vi "SiCellDistMeasure.vi"() -> ()   [LabVIEW 2021]
uses:
  <vilib>/userDefined/High Color/IMAQdx.ctl
  include/GlobalVariables.vi
  Other Models/2010/Motion/AbortSingle.vi
  <vilib>/vision/driver/NI_Vision_Acquisition_Software.lvlib
panel:
  in  "AtEnd":string="G91\nG1 X-12.08 F100\nG90"
  out "error out":errorcluster
  out "XYZdist":string
  out "PrevY":dbl format="%#_13g"
  out "PrevX":dbl format="%#_13g"
  in  "Npoints":i32=14
  in  "NextPosition":string="G91\nG1 X12.08 F100\n//G1 X60.415F100"
  in  "TemplateFileName":string="C:\\Users\\TTUHEP\\Pictures\\Si_Y.png"
  out "CurrXYZdist":string
  in  "ObjectDetType":enum16{"Pattern", "ManualPick", "FidCircle"}(ring)
  in  "StartGCode":string="G90\n//G1 Z0 F100\nG1 X0.7942884\tY965.0350136 F100\rG1 Z75.0089"
  in  "StartPosition":enum16{"JoyStick", "FixedXY"}(ring)
  out "CamY":dbl
  out "CamX":dbl
  out "Radius":dbl
  out "CenterPosition":cluster{"X":sgl, "Y":sgl}
  in  "StopJoyStick":bool
  in  "Autofocus":T1={"Enable"=TRUE, "InitialStepSize"=0.05, "Tolerance"=0.02, "Abort"=FALSE} {"Tolerance" format="%#_13g"}
  out "Image":T2(plugin-control)
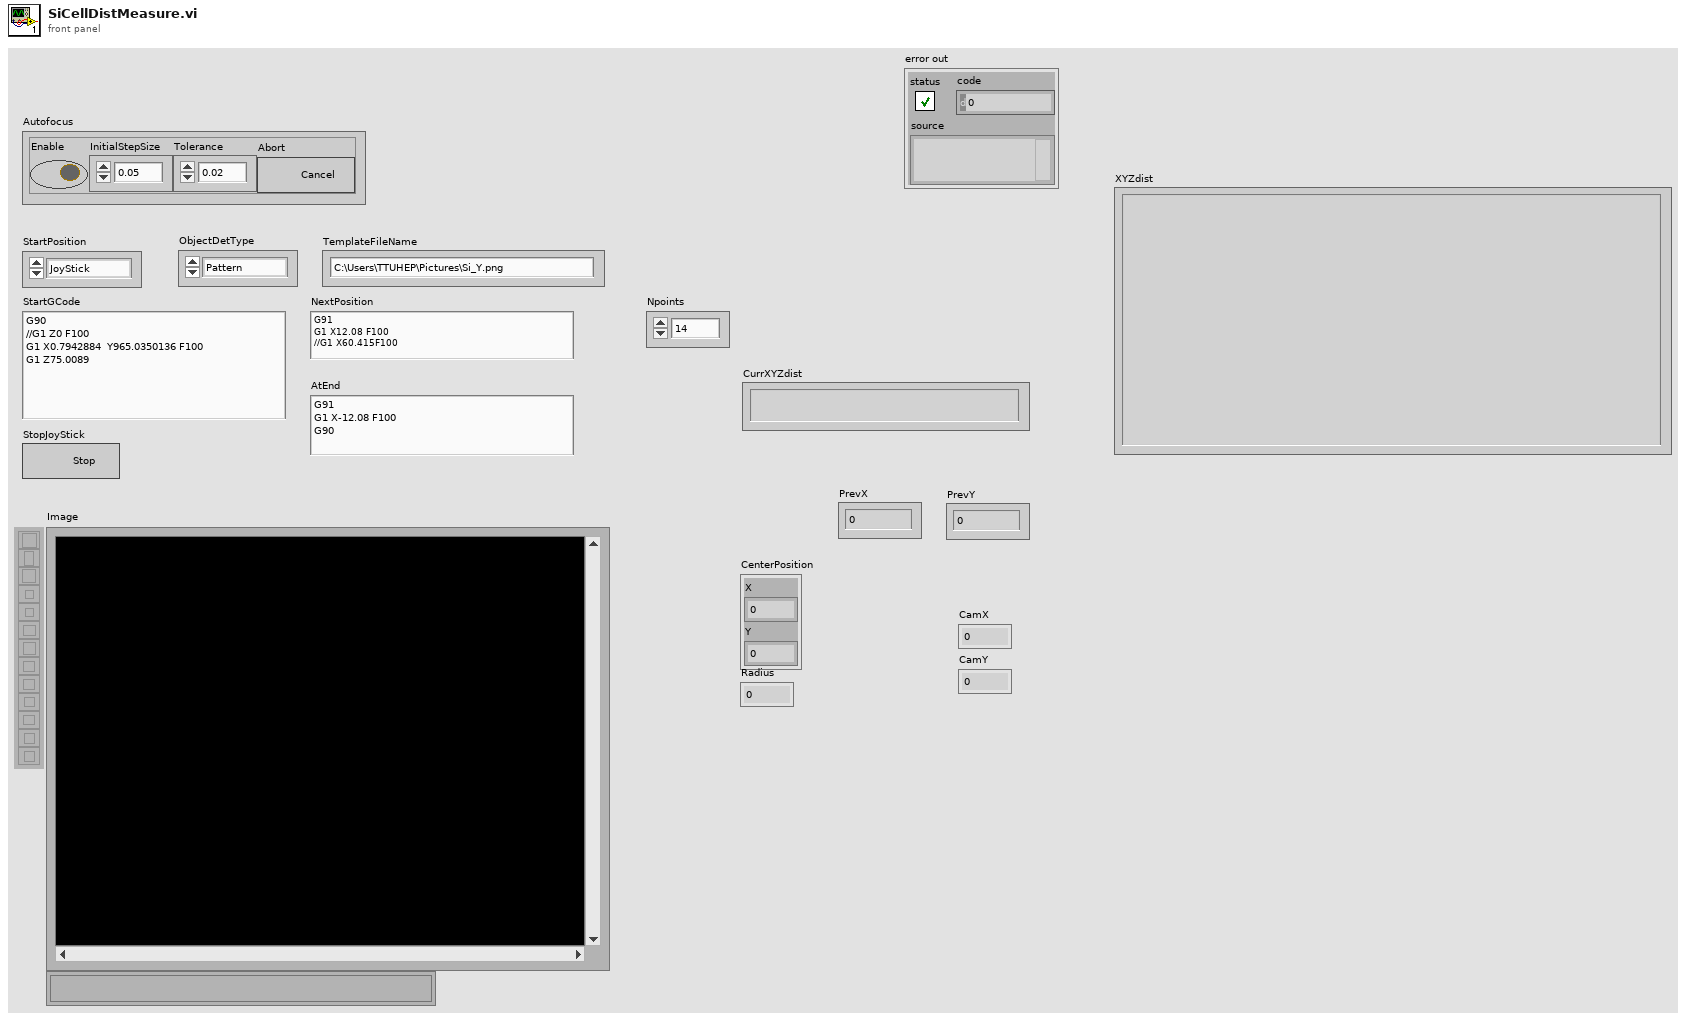
[diagram p1: front panel]
types:
  T1 = cluster{"Enable":bool, "InitialStepSize":dbl, "Tolerance":dbl, "Abort":bool}
  T2 = typedef "IMAQ Image.ctl" = refnum<image>
  T3 = typedef "IMAQdx.ctl" = refnum<k21>
  T4 = typedef "Image Type" = u32
  T5 = cluster{"Number of Matches Requested":i32, "Minimum Match Score":sgl, "Angle Ranges":cluster{"Start Angle":sgl, "End Angle":sgl}[]}
  T6 = typedef "IMAQ Point" = cluster{"X":sgl, "Y":sgl}
  T7 = cluster{"Position":cluster{"X":sgl, "Y":sgl}, "Radius":dbl, "Score":dbl}
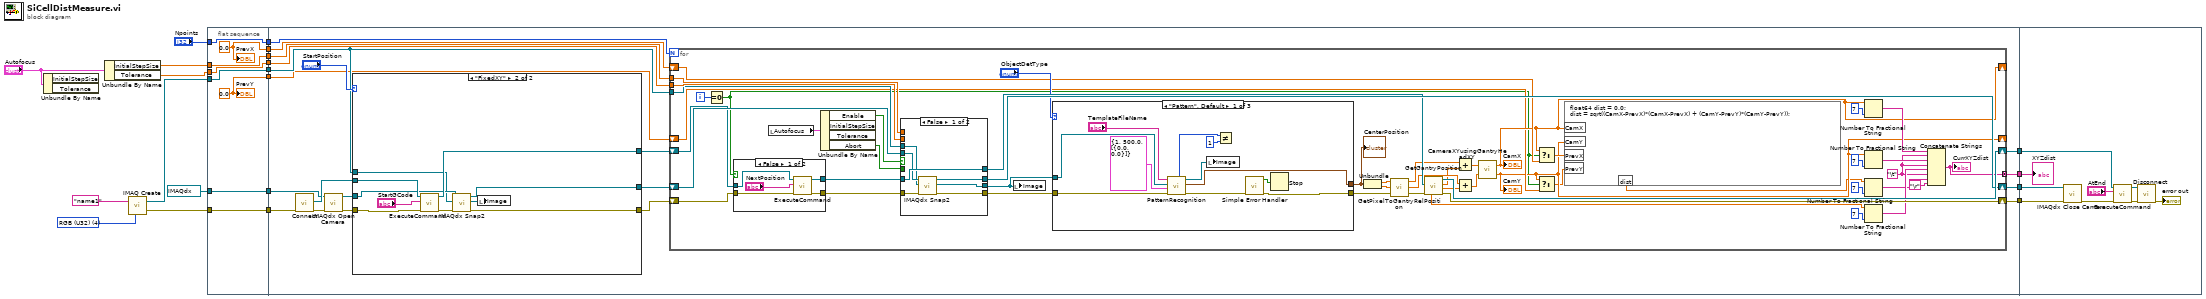
[diagram p0: block diagram]
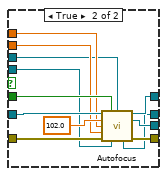
[diagram p3: hidden frame]
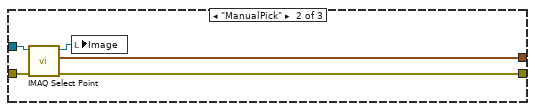
[diagram p4: hidden frame]
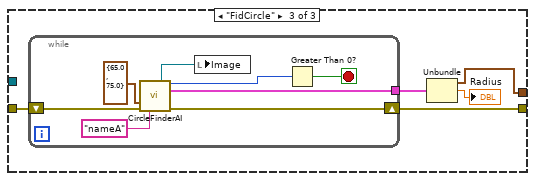
[diagram p5: hidden frame]
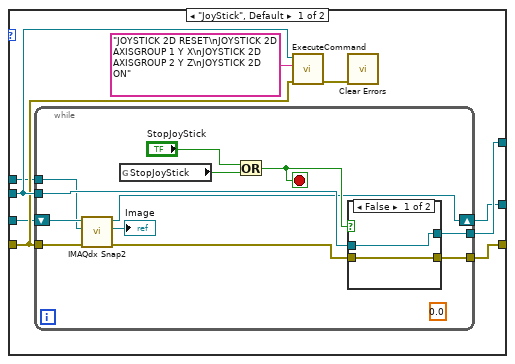
[diagram p6: hidden frame]
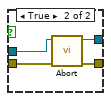
[diagram p7: hidden frame]
diagram:
  w15 = T4 4 items=["Grayscale (U8)", "Grayscale (I16)", "Grayscale (SGL)", "Complex (CSG)", "RGB (U32)", "HSL (U32)", "RGB (U64)", "Grayscale (U16)"] ("Image Type")
  n1 = Unbundle By Name("Autofocus") -> ()  [unwired: 2 out]
  n2 = Unbundle By Name("Autofocus") -> ("InitialStepSize"=w20:dbl, "Tolerance"=w21:dbl)
  n3 = call "IMAQ Create"("Image Name"="name1" ("ImageName"), "Image Type"=w15) -> ("New Image"=w14:T2, "error out"=w13:errorcluster)  [unwired: 3 in]
  n4 = flat-sequence {
    tunnel: "Npoints" -> [w24]
    tunnel: T3 "cam1" ("Camera") -> [w25]
    tunnel: w13 -> [w26]
    tunnel: w14 -> [w27]
    tunnel: w20 -> [w28]
    tunnel: w21 -> [w29]
    tunnel: [w29] -> w9
    tunnel: [w28] -> w8
    tunnel: [w27] -> w7
    tunnel: [w26] -> w6
    tunnel: [w25] -> w5
    tunnel: [w24] -> w4
    tunnel: [w23] -> w3
    tunnel: [w22] -> w2
    tunnel: [w45] -> w18
    tunnel: [w44] -> w17
    tunnel: [w38] -> w11
    tunnel: w9 -> [w49]
    tunnel: w8 -> [w48]
    tunnel: w7 -> [w41]
    tunnel: w6 -> [w42]
    tunnel: w5 -> [w40]
    tunnel: w4 -> [w36]
    tunnel: w3 -> [w33]
    tunnel: w2 -> [w32]
    tunnel: [w31] -> w1
    tunnel: w18 -> [w196]
    tunnel: w17 -> [w200]
    tunnel: w11 -> [w199]
    tunnel: w1 -> [w198]
    frame #0 {
      w22 = 0.0 ("PrevY")
      w23 = 0.0 ("PrevX")
      "PrevX" <- w23
      "PrevY" <- w22
    }
    frame #1 {
      n5 = call "Connect.vi"("error in (no error)"=w42) -> ("error out"=w46:errorcluster, "controller"=w47:refnum<k24>)  [unwired: 9 in]
      n6 = call <vilib>:"IMAQdx Open Camera.vi"("error in"=w46, "Session In"=w40) -> ("error out"=w39:errorcluster, "Session Out"=w30:T3)  [unwired: 8 in]
      n7 = case shown="\"FixedXY\"" "StartPosition" {
        tunnel: w47 -> [w162 w191]
        tunnel: [w160 w189] -> w35
        tunnel: w39 -> [w159 w190]
        tunnel: w41 -> [w158 w183]
        tunnel: w30 -> [w157 w187]
        tunnel: [w156 w185] -> w34
        tunnel: [w155 w184] -> w37
        frame "JoyStick", Default {
          n8 = while {
            tunnel: w162 -> [w175]
            tunnel: [w174] -> w156
            tunnel: [w173] -> w160
            tunnel: w159 -> [w169]
            shift-right: [w167] -> w155
            shift-left: w157 -> [w166]
            tunnel: w158 -> [w164]
            stop <- w170 stop-if-true
            (unwired) sgl 0.0 ("Rotate (degrees)")
            n9 = call <vilib>:"IMAQdx Snap2.vi"("error in"=w169, "Image In"=w164, "Session In"=w166) -> ("error out"=w165:errorcluster, "Image Out"=→"Image":T2, "Session Out"=w167:T3)  [unwired: 6 in]
            n10 = global read "GlobalVariables.vi" "StopJoyStick"() -> (w171:bool)
            n11 = Or(x="StopJoyStick", y=w171) -> (x .or. y?=w170:bool)
            n12 = case shown="False" w170 {
              tunnel: w175 -> [w177 w181]
              tunnel: w165 -> [w176 w180]
              tunnel: [w176 w179] -> w174
              tunnel: [w177 w178] -> w173
              frame False {
              }
              frame True {
                n13 = call-poly "Abort.vi"("error in (no error)"=w180, "controller in"=w181) -> ("error out"=w179:errorcluster, "controller out"=w178:refnum<k24>)  [unwired: 8 in]
              }
            }
          }
          n14 = call "ExecuteCommand.vi"("error in (no error)"=w159, "Command Code"="JOYSTICK 2D RESET\nJOYSTICK 2D AXISGROUP 1 Y X\nJOYSTICK 2D AXISGROUP 2 Y Z\nJOYSTICK 2D ON", "controller in"=w162) -> ("error out"=w161:errorcluster)  [unwired: 6 in, 2 out]
          n15 = call <vilib>:"Clear Errors.vi"("error in (no error)"=w161) -> ()  [unwired: 5 in, 2 out]
        }
        frame "FixedXY" {
          n16 = call "ExecuteCommand.vi"("error in (no error)"=w190, "Command Code"="StartGCode", "controller in"=w191) -> ("error out"=w186:errorcluster, "controller out"=w189:refnum<k24>)  [unwired: 6 in, 1 out]
          n17 = call <vilib>:"IMAQdx Snap2.vi"("error in"=w186, "Image In"=w183, "Session In"=w187) -> ("error out"=w185:errorcluster, "Image Out"=w182:T2, "Session Out"=w184:T3)  [unwired: 6 in]
          n18 = local write "Image"(w182) -> ()
        }
      }
      n19 = for {
        N: w36 -> [_]
        tunnel: w49 -> [w99]
        tunnel: w48 -> [w98]
        tunnel: w41 -> [w89]
        shift-right: [w97] -> w45
        shift-left: w35 -> [w53]
        shift-right: [w96] -> w44
        shift-left: w34 -> [w50]
        shift-right: [w88] -> w38
        shift-left: w37 -> [w71]
        shift-right: [w64] -> _
        shift-left: w33 -> [w65]
        shift-right: [w61] -> _
        shift-left: w32 -> [w63]
        tunnel: [w56] -> w31 mode=concatenating
        i -> [w66]
        w60 = "\t"
        n20 = Equal To 0?(x=w66) -> (x = 0?=w54:bool)
        n21 = case shown="False" w54 {
          tunnel: w53 -> [w103 w105]
          tunnel: [w102 w105] -> w52
          tunnel: [w101 w106] -> w51
          tunnel: w50 -> [w100 w106]
          frame False {
            n22 = call "ExecuteCommand.vi"("error in (no error)"=w100, "Command Code"="NextPosition", "controller in"=w103) -> ("error out"=w101:errorcluster, "controller out"=w102:refnum<k24>)  [unwired: 6 in, 1 out]
          }
          frame True {
          }
        }
        n23 = local read "Autofocus"() -> (w74:T1)
        n24 = Unbundle By Name(w74) -> ("Enable"=w73:bool, "Abort"=w72:bool)  [unwired: 2 out]
        n25 = case shown="False" w73 {
          tunnel: w99 -> [_ w121]
          tunnel: w98 -> [_ w122]
          tunnel: w52 -> [w113 w124]
          tunnel: [w107 w115] -> w87
          tunnel: [w113 w116] -> w86
          tunnel: w51 -> [w108 w120]
          tunnel: [w112 w117] -> w76
          tunnel: w72 -> [_ w125]
          tunnel: w89 -> [w109 w119]
          tunnel: w71 -> [w111 w118]
          tunnel: [w110 w114] -> w88
          frame False {
            n26 = call <vilib>:"IMAQdx Snap2.vi"("error in"=w108, "Image In"=w109, "Session In"=w111) -> ("error out"=w107:errorcluster, "Image Out"=w112:T2, "Session Out"=w110:T3)  [unwired: 6 in]
          }
          frame True {
            n27 = call "Autofocus.vi"("controller in"=w124, "AbortAutoFocus"=w125, "ImageIn"=w119, "SafeMaxZ"=102.0, "InitialStepSize"=w122, "Tolerance"=w121, "error in (no error)"=w120, "SessionIn"=w118) -> ("controller out"=w116:refnum<k24>, "Image"=w117:T2, "Session Out"=w114:T3, "error out"=w115:errorcluster)  [unwired: 2 in, 2 out]
          }
        }
        n28 = local write "Image"(w76) -> ()
        n29 = case shown="\"Pattern\", Default" "ObjectDetType" {
          tunnel: w87 -> [w132 w138 w146]
          tunnel: [w133 w140 w143] -> w85
          tunnel: [w127 w139 w142] -> w82
          tunnel: w76 -> [w135 w141 _]
          frame "Pattern", Default {
            n30 = call "PatternRecognition.vi"("error in (no error)"=w132, "MatchParameters"=T5 {"Number of Matches Requested"=1, "Minimum Match Score"=500.0, "Angle Ranges"=[{"Start Angle"=0.0, "End Angle"=0.0}]}, "ImageIn"=w135, "TemplateFileName"="TemplateFileName") -> ("error out"=w128:errorcluster, "Position"=w133:cluster{"x":sgl, "y":sgl}, "ImageFoundPattern"=w134:T2, "Number of Matches"=w130:i32)  [unwired: 2 in, 1 out]
            n31 = local write "Image"(w134) -> ()
            n32 = Not Equal?(x=w130, y=1) -> ()  [unwired: 1 out]
            n33 = call <vilib>:"Simple Error Handler.vi"("error in (no error)"=w128) -> ("error?"=w126:bool, "error out"=w127:errorcluster)  [unwired: 4 in, 3 out]
            n34 = Stop(stop? (T)=w126) -> ()
          }
          frame "ManualPick" {
            n35 = call "IMAQ Select Point"("error in (no error)"=w138, "Image In"=w141) -> ("error out"=w139:errorcluster, "Point"=w140:T6, "Image Out (duplicate)"=w137:T2)  [unwired: 6 in, 1 out]
            n36 = local write "Image"(w137) -> ()
          }
          frame "FidCircle" {
            n37 = while {
              tunnel: [w151] -> w145
              shift-right: [w150] -> w142
              shift-left: w146 -> [w152]
              stop <- w147 stop-if-true
              n38 = call "CircleFinderAI.vi"("Circle Descriptor"=cluster{"Min Radius":dbl, "Max Radius":dbl} {"Min Radius"=65.0, "Max Radius"=75.0}, "error in (no error)"=w152, "Image Name"="nameA") -> ("Image"=w149:T2, "NumCirclesFound"=w148:i32, "Circle0"=w151:T7, "error out"=w150:errorcluster)  [unwired: 7 in, 2 out]
              n39 = local write "Image"(w149) -> ()
              n40 = Greater Than 0?(x=w148) -> (x > 0?=w147:bool)
            }
            n41 = Unbundle(w145) -> ("Position"=w143:cluster{"X":sgl, "Y":sgl}, "Radius"=→"Radius":dbl)  [unwired: 1 out]
          }
        }
        "CenterPosition" <- w85
        n42 = Unbundle(w85) -> ("X"=w84:sgl, "Y"=w83:sgl)
        n43 = call "GetPixelToGantryRelPosition.vi"("error in (no error)"=w82, "PixelY"=w83, "PixelX"=w84) -> ("error out"=w81:errorcluster, "YmmRelGH"=w79:dbl, "XmmRelGH"=w77:dbl)
        n44 = call "GetGantryPosition.vi"("error in (no error)"=w81, "Controller In"=w86) -> ("error out"=w96:errorcluster, "Position Y"=w80:dbl, "Position X"=w78:dbl, "controller out"=w97:refnum<k24>, "Position Z"=w69:dbl)  [unwired: 3 in, 2 out]
        n45 = Add(x=w77, y=w78) -> (x+y=w94:dbl)
        n46 = Add(x=w79, y=w80) -> (x+y=w92:dbl)
        n47 = call "CameraXYusingGantryHeadXY.vi"("GantryY"=w92, "GantryX"=w94) -> ("CamY"=w61:dbl, "CamX"=w64:dbl)
        "CamX" <- w64
        "CamY" <- w61
        n48 = Select(t=w64, s=w54, f=w65) -> (s? t:f=w62:dbl)
        n49 = Select(t=w61, s=w54, f=w63) -> (s? t:f=w55:dbl)
        n50 = formula code="float64 dist = 0.0;\ndist = sqrt((CamX-PrevX)*(CamX-PrevX) + (CamY-PrevY)*(CamY-PrevY));"("CamX"=w64, "CamY"=w61, "PrevX"=w62, "PrevY"=w55) -> ("dist"=w58:dbl)
        n51 = Number To Fractional String(number=w64, precision (6)=i16 7) -> (F-format string=w91:string)  [unwired: 2 in]
        n52 = Number To Fractional String(number=w61, precision (6)=i16 7) -> (F-format string=w90:string)  [unwired: 2 in]
        n53 = Number To Fractional String(number=w58, precision (6)=i16 7) -> (F-format string=w57:string)  [unwired: 2 in]
        n54 = Number To Fractional String(number=w69, precision (6)=i16 7) -> (F-format string=w68:string)  [unwired: 2 in]
        n55 = Concatenate Strings(w91, w60, w90, w60, w68, w60, w57, "\r") -> (w56:string)
        "CurrXYZdist" <- w56
      }
    }
    frame #2 {
      n56 = call <vilib>:"IMAQdx Close Camera.vi"("error in"=w200, "Session In"=w199) -> ("error out"=w194:errorcluster)  [unwired: 9 in]
      n57 = call "ExecuteCommand.vi"("error in (no error)"=w194, "Command Code"="AtEnd", "controller in"=w196) -> ("error out"=w193:errorcluster, "controller out"=w192:refnum<k24>)  [unwired: 6 in, 1 out]
      n58 = call "Disconnect.vi"("error in (no error)"=w193, "controller"=w192) -> ("error out"=→"error out":errorcluster)  [unwired: 9 in]
      "XYZdist" <- w198
    }
  }
